vi "WPI_DashboardSeek to Scrub Time2.vi"(6 "Docked Window":bool, 8 "VI Refnum":refnum<vi>, 9 "latest update tick":timestamp, 10 "TimeOffset (s)":dbl, 11 "Byte Stream File in":refnum<file>) -> (0 "Strings":T1, 1 "ms tick out":timestamp, 2 "TimeOffset (s) out":dbl, 3 "Byte Stream File out":refnum<file>)   [LabVIEW 2017]
uses:
  <vilib>/Rock Robotics/WPI/Dashboard/WPI_DashboardNTL Header Type.ctl
  <vilib>/Rock Robotics/WPI/Dashboard/WPI_DashboardPlay Operation.ctl
  <vilib>/Rock Robotics/WPI/Dashboard/WPI_DashboardLogging Global.vi
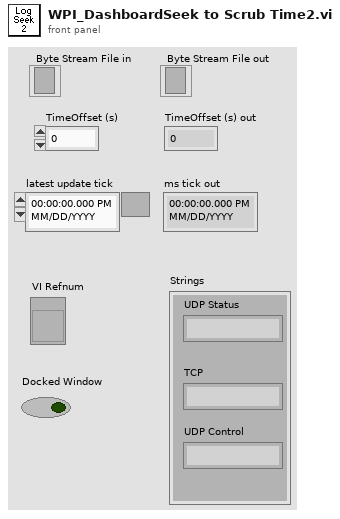
[diagram p1: front panel]
types:
  T1 = cluster{"UDP Status":string, "TCP":string, "UDP Control":string}
  T2 = typedef "WPI_DashboardPlay Operation.ctl" = enum16{"Play", "Pause", "Finished"}
  T3 = typedef "WPI_DashboardNTL Header Type.ctl" = cluster{"Version":i32, "Duration (ms)":i32, "TimeStamp":timestamp, "Robot IP":string, "Displays":string[]}
  T4 = enum16{"1/10", "1/5", "1/2", "1", "2", "5", "10"}
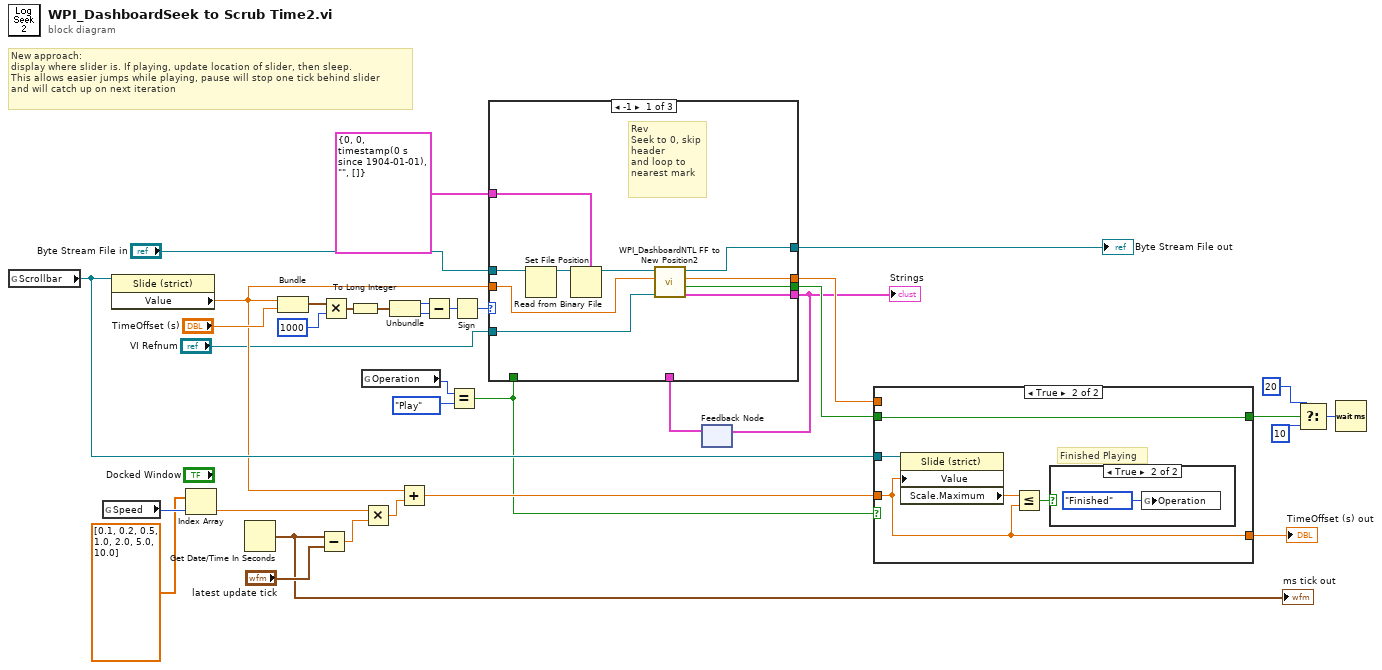
[diagram p0: block diagram]
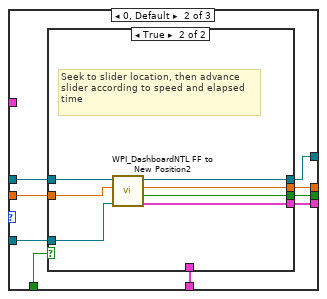
[diagram p4: hidden frame]
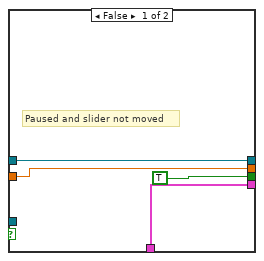
[diagram p5: hidden frame]
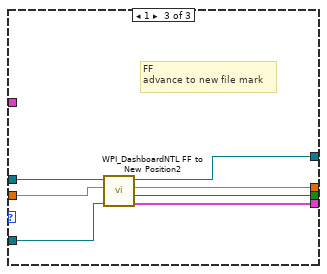
[diagram p6: hidden frame]
diagram:
  # "New approach:\ndisplay where slider is. If playing, update location of slider, then sleep.\nThis allows easier jumps while playing, pause will stop one tick behind slider\nand will catch up on next iteration"
  n1 = global read "WPI_DashboardLogging Global.vi" "Scrollbar"() -> (w16:refnum<vi>)
  n2 = global read "WPI_DashboardLogging Global.vi" "Speed"() -> (w30:T4)
  n3 = property class="Slide (strict)"(reference=w16) -> ("Value"=w4:dbl)  [unwired: 1 in, 2 out]
  n4 = Index Array(array=dbl[] [0.1, 0.2, 0.5, 1.0, 2.0, 5.0, 10.0], index=w30) -> (element=w28:dbl)
  n5 = Get Date/Time In Seconds() -> (seconds since 1Jan1904=w7:timestamp)
  "ms tick out" <- w7
  n6 = Bundle("Value"=w4, "TimeOffset (s)"="TimeOffset (s)") -> (w20:cluster{"Value":dbl, "TimeOffset (s)":dbl})  [unwired: 1 in]
  n7 = Subtract(x=w7, y="latest update tick") -> (x-y=w27:dbl)
  n8 = Multiply(x=w20, y=1000) -> (x*y=w21:cluster{"Value":dbl, "TimeOffset (s)":dbl})
  n9 = To Long Integer(number=w21) -> (32bit integer=w19:cluster{"Value":i32, "TimeOffset (s)":i32})
  n10 = global read "WPI_DashboardLogging Global.vi" "Operation"() -> (w17:T2)
  n11 = Multiply(x=w28, y=w27) -> (x*y=w15:dbl)
  n12 = Unbundle(w19) -> ("Value"=w23:i32, "TimeOffset (s)"=w22:i32)
  n13 = Add(x=w4, y=w15) -> (x+y=w12:dbl)
  n14 = Subtract(x=w23, y=w22) -> (x-y=w32:i32)
  n15 = Equal?(x=w17, y=WPI_DashboardPlay_Operation."Play" ("Operation")) -> (x = y?=w8:bool)
  n16 = Sign(1:w32) -> (0:w33:i32)
  n17 = feedback #1() -> (w3:T1)  [unwired: 1 in]
  n18 = case shown="-1" w33 {
    tunnel: "Byte Stream File in" -> [w45 w54 w72]
    tunnel: [w40 w53 w70] -> w35
    tunnel: T3 {"Version"=0, "Duration (ms)"=0, "TimeStamp"=timestamp(0 s since 1904-01-01), "Robot IP"="", "Displays"=[]} ("Header") -> [w43 _ _]
    tunnel: w4 -> [w36 w50 w71]
    tunnel: [w39 w52 w69] -> w14
    tunnel: [w41 w51 w68] -> w10
    tunnel: w8 -> [_ w49 _]
    tunnel: [w42 w48 w66] -> w1
    tunnel: w3 -> [_ w47 _]
    tunnel: "VI Refnum" -> [w37 w46 w67]
    frame -1 {
      # "Rev\nSeek to 0, skip\nheader\nand loop to\nnearest mark"
      n19 = Set File Position(refnum=w45) -> (refnum out=w44:refnum<file>)  [unwired: 3 in, 1 out]
      n20 = Read from Binary File(5:w43, 11:w44) -> (3:w38:refnum<file>)  [unwired: 4 in, 3 out]
      n21 = call <vilib>:"WPI_DashboardNTL FF to New Position2.vi"("VI Refnum"=w37, "TimeOffset (s)"=w36, "Byte Stream File in"=w38) -> ("Strings"=w42:T1, "Unchanged"=w41:bool, "New time (s)"=w39:dbl, "Byte Stream File out"=w40:refnum<file>)  [unwired: 5 in]
    }
    frame 0, Default {
      n22 = case shown="True" w49 {
        tunnel: w54 -> [w58 w65]
        tunnel: [w58 w62] -> w53
        tunnel: [w56 w61] -> w52
        tunnel: [TRUE w60] -> w51
        tunnel: w50 -> [w56 w64]
        tunnel: [w55 w59] -> w48
        tunnel: w47 -> [w55 _]
        tunnel: w46 -> [_ w63]
        frame False {
          # "Paused and slider not moved"
        }
        frame True {
          # "Seek to slider location, then advance\nslider according to speed and elapsed\ntime"
          n23 = call <vilib>:"WPI_DashboardNTL FF to New Position2.vi"("VI Refnum"=w63, "TimeOffset (s)"=w64, "Byte Stream File in"=w65) -> ("Strings"=w59:T1, "Unchanged"=w60:bool, "New time (s)"=w61:dbl, "Byte Stream File out"=w62:refnum<file>)  [unwired: 5 in]
        }
      }
    }
    frame 1 {
      # "FF\nadvance to new file mark"
      n24 = call <vilib>:"WPI_DashboardNTL FF to New Position2.vi"("VI Refnum"=w67, "TimeOffset (s)"=w71, "Byte Stream File in"=w72) -> ("Strings"=w66:T1, "Unchanged"=w68:bool, "New time (s)"=w69:dbl, "Byte Stream File out"=w70:refnum<file>)  [unwired: 5 in]
    }
  }
  "Byte Stream File out" <- w35
  "Strings" <- w1
  n25 = feedback-in #1(w1) -> ()
  n26 = case shown="True" w8 {
    tunnel: w16 -> [_ w79]
    tunnel: w14 -> [w74 _]
    tunnel: w12 -> [_ w76]
    tunnel: [w74 w76] -> w13
    tunnel: [w73 w78] -> w9
    tunnel: w10 -> [w73 w78]
    frame False {
    }
    frame True {
      # "Finished Playing"
      n27 = property class="Slide (strict)"(reference=w79, "Value"=w76) -> ("Scale.Maximum"=w77:dbl)  [unwired: 1 in, 2 out]
      n28 = Less Or Equal?(x=w77, y=w76) -> (x <= y?=w75:bool)
      n29 = case shown="True" w75 {
        frame False {
        }
        frame True {
          n30 = global write "WPI_DashboardLogging Global.vi" "Operation"(WPI_DashboardPlay_Operation."Finished" ("Operation")) -> ()
        }
      }
    }
  }
  "TimeOffset (s) out" <- w13
  n31 = Select(t=20, s=w9, f=10) -> (s? t:f=w26:i32)
  n32 = Wait (ms)(milliseconds to wait=w26) -> ()  [unwired: 1 out]
